vi "_extractWaveformProperties - Copy.vi"(0 "Waveforms":waveform(dbl)[](array[waveform]), 1 "Property Values":variant[][](array[variant]), 2 "Property Names":string[][](array[string]), 5 "File Name":string, 7 "Channel Names":string[](array[string]), 9 "Group Name":string, 11 "error in (no error)":errorcluster) -> (4 "Event Object":string[](array[string]), 6 "Starting Index Increment":u32[](array[numeric]), 15 "error out":errorcluster)   [LabVIEW 2019]
uses:
  f393d158-72fd-4f86-9db4-308c5760cb49.vi
  9ed0ff8f-8473-4484-9245-6b3cf206dcee.vi
  134c6dd0-6cc6-4c6e-a78f-761504b1249a.vi
  9ef9f007-351d-46b5-8410-71036a852954.vi
  <vilib>/JDP Science/JSONtext/support/Format JSON Object.vi
  <vilib>/JDP Science/JSONtext/JSONtext.lvlib
  <vilib>/Utility/Data Type/NI_Data Type.lvlib
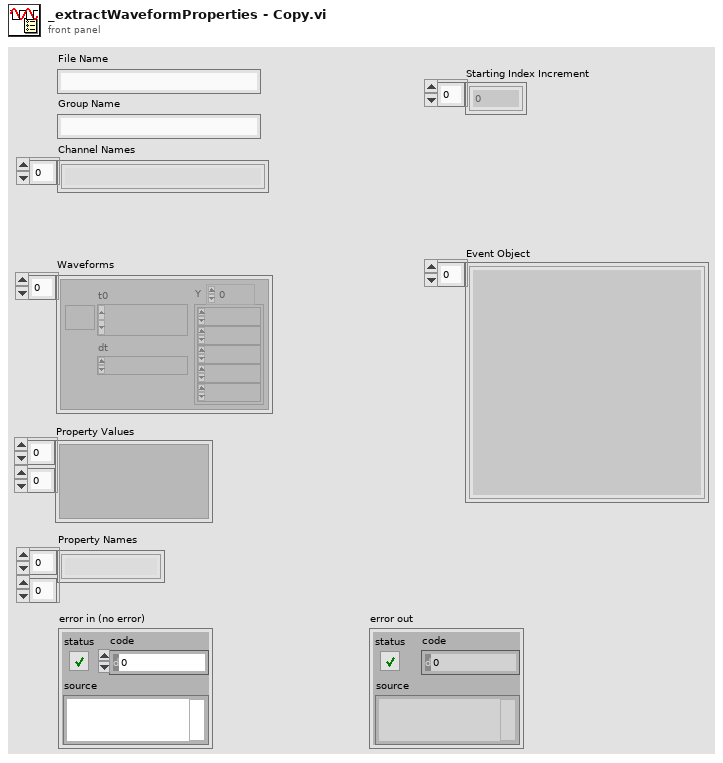
[diagram p1: front panel]
types:
  T1 = typedef "NI_Data Type.lvlib/Data Type.ctl" = enum8{"Invalid Type", "Void", "I8", "I16", "I32", "I64", "U8", "U16", "U32", "U64", "Single Float", "Double Float", "Extended Float", "Single Complex", "Double Complex", "Extended Complex", "Enum U8", "Enum U16", "Enum U32", "Enum U64", "Single Float With Unit", "Double Float With Unit", "Extended Float With Unit", "Single Complex with Unit", "Double Complex with Unit", "Extended Complex with Unit", "Boolean", "String", "Path", "Picture", "Tag", "Array", "Cluster", "Variant", "LV Variant", "Waveform", "Timestamp", "Digital Waveform", "Digital Data", "ExpressData", "Refnum", "External Data", "VI", "Poly VI", "LabVIEW Class Instance", "Fixed Point", "Set Collection", "Map Collection"}
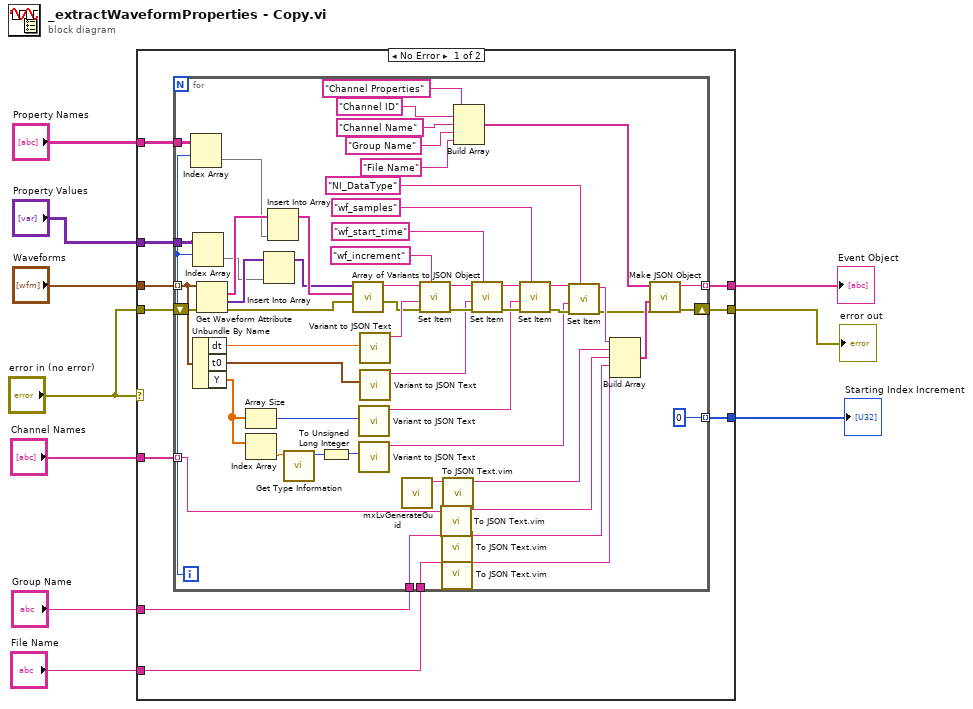
[diagram p0: block diagram]
diagram:
  n1 = case shown="No Error" "error in (no error)" {
    selector: "error in (no error)" -> [_ w76]
    tunnel: "Waveforms" -> [w20 _]
    tunnel: "error in (no error)" -> [w19 _]
    tunnel: [w18 w76] -> w8
    tunnel: [w17 _] -> w7
    tunnel: "Channel Names" -> [w16 _]
    tunnel: "Group Name" -> [w15 _]
    tunnel: "File Name" -> [w14 _]
    tunnel: [w13 _] -> w3
    tunnel: "Property Names" -> [w12 _]
    tunnel: "Property Values" -> [w11 _]
    frame No Error {
      n2 = for {
        tunnel: w20 -> [w73] mode=indexing
        shift-right: [w58] -> w18
        shift-left: w19 -> [w75]
        tunnel: [w54] -> w17 mode=indexing
        tunnel: w16 -> [w50] mode=indexing
        tunnel: w15 -> [w48]
        tunnel: w14 -> [w47]
        tunnel: [u32 0] -> w13 mode=indexing
        tunnel: w12 -> [w25]
        tunnel: w11 -> [w23]
        i -> [w21]
        n3 = Index Array(array=w25, index (row)=w21) -> (element=w24:string[])  [unwired: 1 in]
        n4 = Index Array(array=w23, index (row)=w21) -> (element=w22:variant[])  [unwired: 1 in]
        n5 = Unbundle By Name(w73) -> ("dt"=w72:dbl, "t0"=w71:timestamp, "Y"=w35:dbl[])
        n6 = Get Waveform Attribute(4:w75, 7:w73) -> (0:w74:errorcluster, 1:w27:variant[], 2:w29:string[])  [unwired: 2 in, 1 out]
        n7 = Array Size(array=w35) -> (size(s)=w41:i32)
        n8 = Index Array(array=w35) -> (element=w34:dbl)  [unwired: 1 in]
        n9 = Insert Into Array(array=w27, new element=w22) -> (w26:variant[])  [unwired: 1 in]
        n10 = Insert Into Array(array=w29, new element=w24) -> (w28:string[])  [unwired: 1 in]
        n11 = call <vilib>:"Get Type Information.vi"("variant"=w34) -> ("type"=w33:T1)  [unwired: 6 in, 4 out]
        n12 = To Unsigned Long Integer(number=w33) -> (unsigned 32bit integer=w32:u32)
        n13 = call <vilib>:"Array of Variants to JSON Object.vi"("error in (no error)"=w74, "Names"=w28, "Array"=w26) -> ("error out"=w59:errorcluster, "<JSON>"=w60:string)  [unwired: 7 in]
        n14 = call <vilib>:"Variant to JSON Text.vi"("Variant"=w41) -> ("<JSON>"=w62:string)  [unwired: 8 in, 2 out]
        n15 = call <vilib>:"Variant to JSON Text.vi"("Variant"=w32) -> ("<JSON>"=w31:string)  [unwired: 8 in, 2 out]
        n16 = call <vilib>:"Variant to JSON Text.vi"("Variant"=w72) -> ("<JSON>"=w61:string)  [unwired: 8 in, 2 out]
        n17 = call <vilib>:"Variant to JSON Text.vi"("Variant"=w71) -> ("<JSON>"=w67:string)  [unwired: 8 in, 2 out]
        n18 = call <resource>:"mxLvGenerateGuid.vi"() -> ("Value"=w44:string)  [unwired: 10 in, 1 out]
        n19 = call <vilib>:"Set Item.vi"("$Path or Item Name"="wf_increment", "error in (no error)"=w59, "JSON to Insert"=w61, "JSON"=w60) -> ("error out"=w68:errorcluster, "<JSON>"=w69:string)  [unwired: 4 in, 1 out]
        n20 = call "To JSON Text.vim"("Anything"=w50) -> ("<JSON>"=w49:string)  [unwired: 9 in, 1 out]
        n21 = call "To JSON Text.vim"("Anything"=w48) -> ("<JSON>"=w46:string)  [unwired: 9 in, 1 out]
        n22 = call "To JSON Text.vim"("Anything"=w47) -> ("<JSON>"=w45:string)  [unwired: 9 in, 1 out]
        n23 = call "To JSON Text.vim"("Anything"=w44) -> ("<JSON>"=w43:string)  [unwired: 9 in, 1 out]
        n24 = Build Array("Channel Properties" ("$Path or Item Name"), "Channel ID" ("element"), "Channel Name" ("$Path or Item Name"), "Group Name" ("$Path or Item Name"), "File Name" ("$Path or Item Name")) -> (w56:string[])
        n25 = call <vilib>:"Set Item.vi"("$Path or Item Name"="wf_start_time", "error in (no error)"=w68, "JSON to Insert"=w67, "JSON"=w69) -> ("error out"=w65:errorcluster, "<JSON>"=w64:string)  [unwired: 4 in, 1 out]
        n26 = call <vilib>:"Set Item.vi"("$Path or Item Name"="wf_samples", "error in (no error)"=w65, "JSON to Insert"=w62, "JSON"=w64) -> ("error out"=w36:errorcluster, "<JSON>"=w39:string)  [unwired: 4 in, 1 out]
        n27 = call <vilib>:"Set Item.vi"("$Path or Item Name"="NI_DataType", "error in (no error)"=w36, "JSON to Insert"=w31, "JSON"=w39) -> ("error out"=w37:errorcluster, "<JSON>"=w38:string)  [unwired: 4 in, 1 out]
        n28 = Build Array(w38, w43, w49, w46, w45) -> (w55:string[])
        n29 = call <vilib>:"Make JSON Object.vi"("error in (no error)"=w37, "JSON Items"=w55, "Item Names"=w56) -> ("error out"=w58:errorcluster, "<JSON>"=w54:string)  [unwired: 7 in]
      }
    }
    frame Error {
    }
  }
  "error out" <- w8
  "Event Object" <- w7
  "Starting Index Increment" <- w3
